vi "Playground.vi"(11 "Inset":refnum<class "Inset.lvclass">) -> (3 "Inset out":refnum<class "Inset.lvclass">)   [LabVIEW 2019, in "Inset.lvclass"]
uses:
  Inset.lvclass
  Parse/Image/SVGImage.lvclass
  C:/Users/Albro/Documents/GitHub/AFM-Lithography/lvsrc/Classes/Parse/SVG Object/SVG Object.lvclass
  Parse/ParseXML/ParseSVG.lvclass
  Parse/ParseVectorFile/ParseVectorFile.lvclass
  Parse/ParseXML/Image.ctl
  Parse/ParseXML/ParseSVG.lvclass/ParseSVG.ctl
  <vilib>/LabVIEW Open Source Project/OpenURI/utilities/isHEXDigit.vi
  BigMAQ/BigMAQ.lvclass
  Parse/EditSVG/EditSVG.lvclass
  <vilib>/LabVIEW Open Source Project/OpenURI/openURI.lvlib
panel:
  out "Pct-Encoded String":string
  out "Edited XML":string
  out "BGD Size":dbl
  out "Y Offset 2":string
  out "ScanSize 2":string
  out "BGD Y Offset":dbl
  out "BGD X Offset":dbl
  out "Inset X Offset":dbl
  out "Inset Y Offset":dbl
  out "Inset Size":dbl
  out "SVGImage.lvclass":refnum<class "SVGImage.lvclass">
  out "ScanSize":string
  out "Y Offset":string
  in  "Inkscape Path":path
  in  "Background Path":path=path "C:/Users/Albro/Documents/GitHub/AFM-Lithography/test files/Inset Test Files/R_tMLG_Au0003.ibw"
  in  "Inset Path":path=path "C:/Users/Albro/Documents/GitHub/AFM-Lithography/test files/Inset Test Files/R_tMLG_Au0004.ibw"
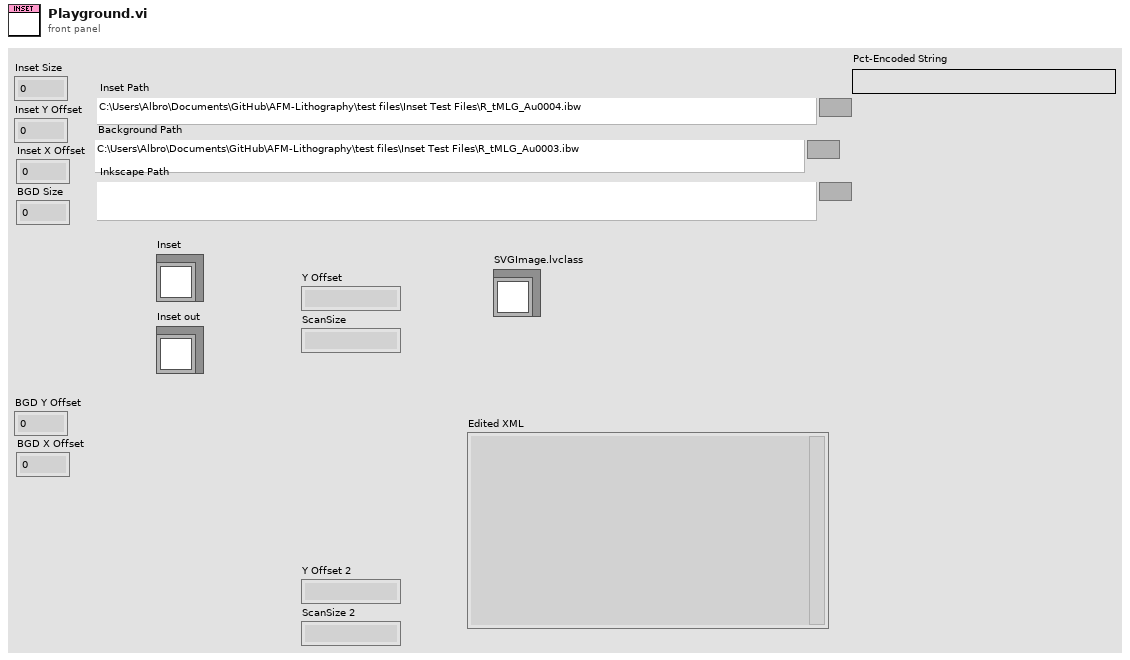
[diagram p1: front panel]
types:
  T1 = cluster{"Inkscape":path, "Background":path, "Inset":path}
  T2 = typedef "ParseSVG.lvclass/Image.ctl" = cluster{"x":string, "y":string, "width":string, "height":string, "xlink:href":string, "id":string, "transform":string}
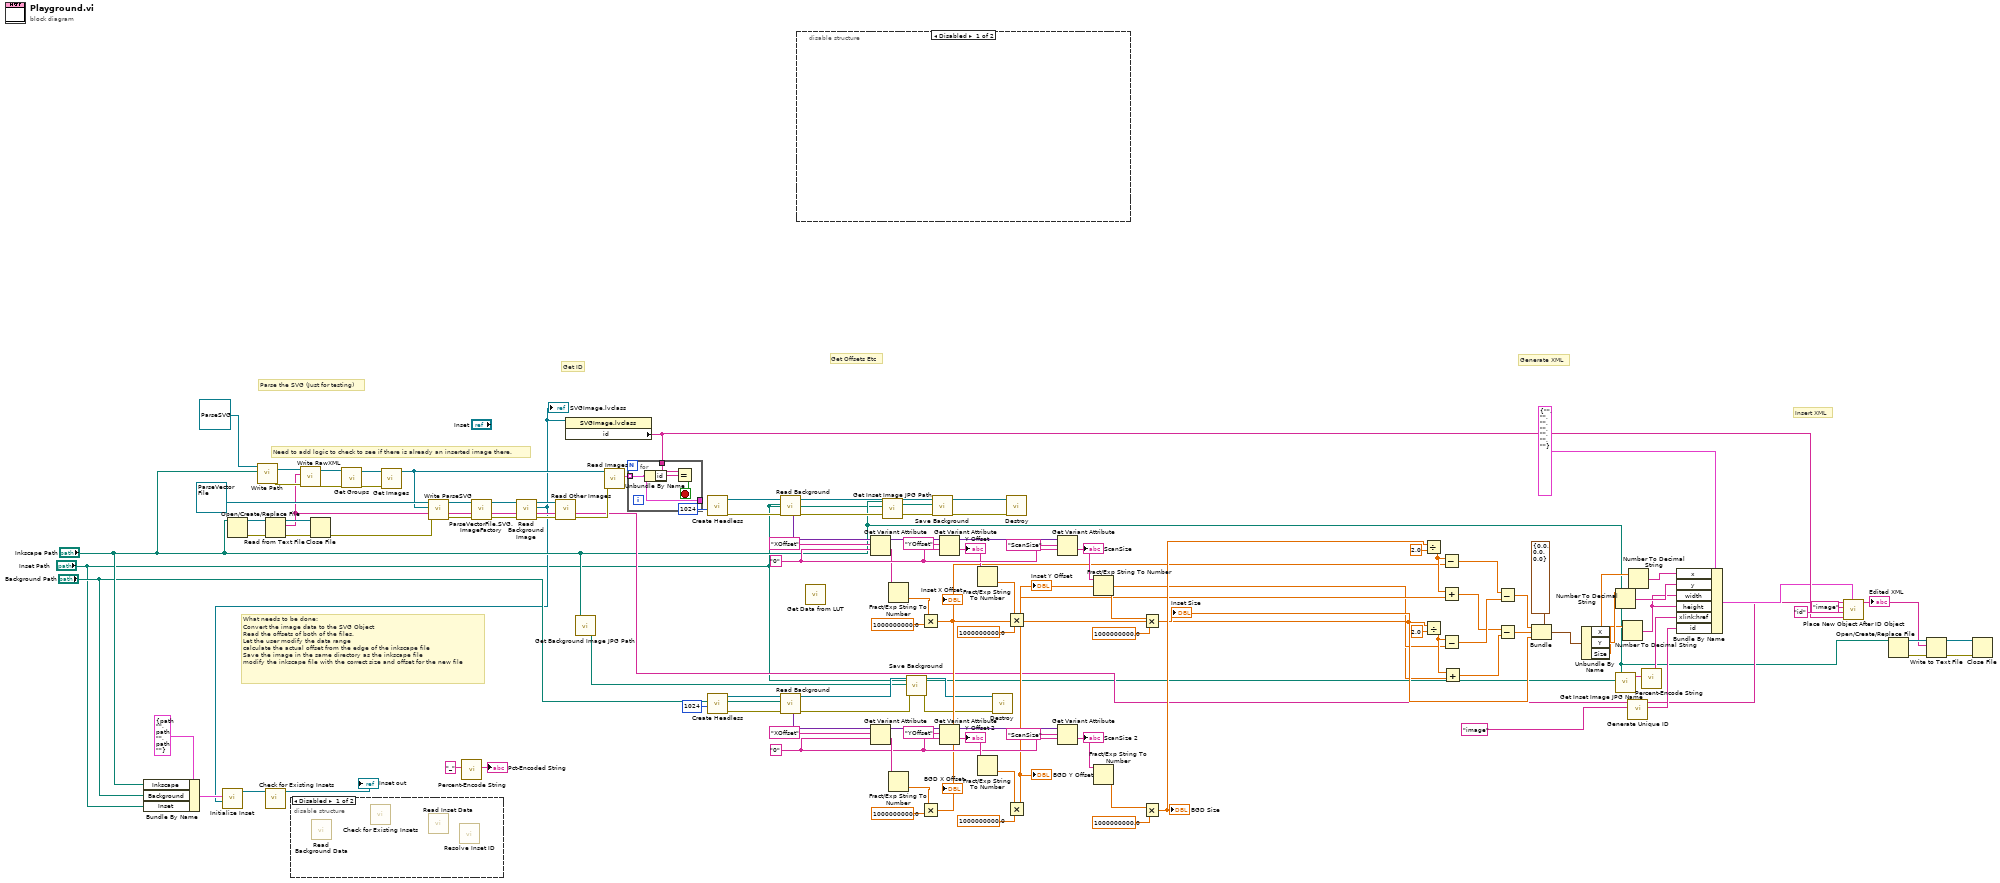
[diagram p0: block diagram]
diagram:
  w66 = "0"
  w114 = "0"
  # "Parse the SVG (Just for testing)"
  # "Insert XML"
  # "Generate XML"
  # "Get Offsets Etc"
  # "Get ID"
  # "Need to add logic to check to see if there is already an inserted image there."
  # "What needs to be done:\nConvert the image data to the SVG Object\nRead the offsets of both of the files.\nLet the user modify the data range\ncalculate the actual offset from the edge of the inkscape file\nSave the image in the same directory as the inkscape file\nmodify the inkscape file with the correct size and offset for the new file"
  n1 = Bundle By Name(cluster=T1 {"Inkscape"=path "", "Background"=path "", "Inset"=path ""} ("Paths"), "Inkscape"="Inkscape Path", "Background"="Background Path", "Inset"="Inset Path") -> (w11:T1)
  n2 = Open/Create/Replace File(file path (use dialog)="Inkscape Path") -> (refnum out=w103:refnum<file>, error out=w101:errorcluster)  [unwired: 5 in, 1 out]
  n3 = call-dynamic "Write Path.vi"("Path"="Inkscape Path", "ParseSVG in"=refnum<class "ParseSVG.lvclass"> refnum) -> ("error out"=w111:errorcluster, "ParseSVG out"=w112:refnum<class "ParseSVG.lvclass">)  [unwired: 8 in]
  n4 = Read from Text File(file (use dialog)=w103, error in=w101) -> (refnum out=w102:refnum<file>, text=w17:string, error out=w100:errorcluster)  [unwired: 2 in, 1 out]
  n5 = disable-structure shown="Disabled" {
    frame Disabled {
      n6 = call "Read Background Data.vi"() -> ()  [unwired: 10 in, 2 out]
      n7 = call "Check for Existing Insets.vi"() -> ()  [unwired: 10 in, 2 out]
      n8 = call "Read Inset Data.vi"() -> ()  [unwired: 10 in, 2 out]
      n9 = call "Resolve Inset ID.vi"() -> ()  [unwired: 10 in, 2 out]
    }
    frame Enabled {
    }
  }
  n10 = call "Write RawXML.vi"("error in (no error)"=w111, "RawXML"=w17, "ParseSVG.lvclass"=w112) -> ("error out"=w109:errorcluster, "ParseSVG.lvclass 2"=w110:refnum<class "ParseSVG.lvclass">)  [unwired: 7 in]
  n11 = Close File(refnum=w102, error in=w100) -> (error out=w99:errorcluster)  [unwired: 1 out]
  n12 = call "Get Groups.vi"("error in (no error)"=w109, "ParseSVG in"=w110) -> ("error out"=w107:errorcluster, "ParseSVG out"=w108:refnum<class "ParseSVG.lvclass">)  [unwired: 8 in]
  n13 = call "Get Images.vi"("error in (no error)"=w107, "ParseSVG in"=w108) -> ("ParseSVG out"=w93:refnum<class "ParseSVG.lvclass">)  [unwired: 8 in, 1 out]
  n14 = call-dynamic "Write ParseSVG.vi"("error in (no error)"=w99, "ParseSVG.lvclass"=w93, "ParseVectorFile in"=refnum<class "ParseVectorFile.lvclass"> refnum ("ParseVectorFile.lvclass")) -> ("error out"=w104:errorcluster, "ParseVectorFile out"=w105:refnum<class "ParseVectorFile.lvclass">)  [unwired: 7 in]
  n15 = call <vilib>:"Percent-Encode String.vi"("String"="_") -> ("Pct-Encoded String"=→"Pct-Encoded String":string)  [unwired: 10 in]
  n16 = call "ParseVectorFile.SVG.ImageFactory.vi"("error in (no error)"=w104, "ParseVectorFile in"=w105) -> ("error out"=w97:errorcluster, "ParseVectorFile out"=w98:refnum<class "ParseVectorFile.lvclass">)  [unwired: 8 in]
  n17 = call-dynamic "Read Background Image.vi"("error in (no error)"=w97, "ParseVectorFile in"=w98) -> ("error out"=w95:errorcluster, "SVGImage.lvclass"=w8:refnum<class "SVGImage.lvclass">, "ParseVectorFile out"=w96:refnum<class "ParseVectorFile.lvclass">)  [unwired: 7 in]
  "SVGImage.lvclass" <- w8
  n18 = call "Initialize Inset.vi"("Background Image"=w8, "Paths"=w11) -> ("Inset out"=w4:refnum<class "Inset.lvclass">)  [unwired: 8 in, 1 out]
  n19 = call "Check for Existing Insets.vi"("Inset in"=w4) -> ("Inset out"=→"Inset out":refnum<class "Inset.lvclass">)  [unwired: 9 in, 1 out]
  n20 = call-dynamic "Read Other Images.vi"("error in (no error)"=w95, "ParseVectorFile in"=w96) -> ("error out"=w94:errorcluster)  [unwired: 7 in, 2 out]
  n21 = property class="SVGImage.lvclass"(reference=w8) -> ("id"=w26:string)  [unwired: 1 in, 2 out]
  n22 = call "Get Background Image JPG Path.vi"("Inkscape Path"="Inkscape Path") -> ("Background JPG Path"=w13:path)  [unwired: 2 in]
  n23 = call "Read Images.vi"("error in (no error)"=w94, "ParseSVG in"=w93) -> ("Images"=w92:T2[])  [unwired: 7 in, 2 out]
  n24 = for {
    tunnel: w92 -> [w120] mode=indexing
    tunnel: w26 -> [w122]
    tunnel: [w120] -> _
    stop <- w121 stop-if-true
    n25 = Unbundle By Name(w120) -> ("id"=w123:string)
    n26 = Equal?(x=w122, y=w123) -> (x = y?=w121:bool)
  }
  n27 = call "Create Headless.vi"("Resolution"=1024) -> ("error out"=w89:errorcluster, "BigMAQ out"=w90:refnum<class "BigMAQ.lvclass">)  [unwired: 9 in]
  n28 = call "Create Headless.vi"("Resolution"=1024) -> ("error out"=w77:errorcluster, "BigMAQ out"=w78:refnum<class "BigMAQ.lvclass">)  [unwired: 9 in]
  n29 = call "Read Background.vi"("error in (no error)"=w89, "Path"="Inset Path", "BigMAQ in"=w90) -> ("error out"=w56:errorcluster, "BigMAQ out"=w59:refnum<class "BigMAQ.lvclass">, "Metadata"=w88:variant)  [unwired: 6 in]
  n30 = call "Read Background.vi"("error in (no error)"=w77, "Path"="Background Path", "BigMAQ in"=w78) -> ("error out"=w14:errorcluster, "BigMAQ out"=w16:refnum<class "BigMAQ.lvclass">, "Metadata"=w60:variant)  [unwired: 6 in]
  n31 = disable-structure shown="Disabled" {
    frame Disabled {
    }
    frame Enabled {
    }
  }
  n32 = call "Get Data from LUT.vi"() -> ()  [unwired: 9 in, 3 out]
  n33 = Get Variant Attribute(Variant=w88, name="XOffset", default value (empty Variant)=w114) -> (duplicate Variant=w118:variant, value=w85:string)  [unwired: 1 in, 2 out]
  n34 = Get Variant Attribute(Variant=w60, name="XOffset", default value (empty Variant)=w66) -> (duplicate Variant=w62:variant, value=w69:string)  [unwired: 1 in, 2 out]
  n35 = call "Get Inset Image JPG Path.vi"("Inset Data Path"="Inset Path", "Inkscape Path"="Inkscape Path") -> ("Inset JPG Path"=w57:path)  [unwired: 3 in]
  n36 = Fract/Exp String To Number(string=w85) -> (number=w84:dbl)  [unwired: 3 in, 1 out]
  n37 = Fract/Exp String To Number(string=w69) -> (number=w70:dbl)  [unwired: 3 in, 1 out]
  n38 = call "Save Background.vi"("error in"=w14, "File Path"=w13, "BigMAQ in"=w16) -> ("error out"=w6:errorcluster, "BigMAQ out"=w15:refnum<class "BigMAQ.lvclass">)  [unwired: 7 in]
  n39 = Multiply(x=w84, y=1000000000.0) -> (x*y=w41:dbl)
  "Inset X Offset" <- w41
  n40 = Multiply(x=w70, y=1000000000.0) -> (x*y=w44:dbl)
  "BGD X Offset" <- w44
  n41 = call "Save Background.vi"("error in"=w56, "File Path"=w57, "BigMAQ in"=w59) -> ("error out"=w7:errorcluster, "BigMAQ out"=w58:refnum<class "BigMAQ.lvclass">)  [unwired: 7 in]
  n42 = Get Variant Attribute(Variant=w118, name="YOffset", default value (empty Variant)=w114) -> (duplicate Variant=w116:variant, value=w86:string)  [unwired: 1 in, 2 out]
  "Y Offset" <- w86
  n43 = Get Variant Attribute(Variant=w62, name="YOffset", default value (empty Variant)=w66) -> (duplicate Variant=w64:variant, value=w68:string)  [unwired: 1 in, 2 out]
  "Y Offset 2" <- w68
  n44 = Fract/Exp String To Number(string=w86) -> (number=w81:dbl)  [unwired: 3 in, 1 out]
  n45 = Fract/Exp String To Number(string=w68) -> (number=w73:dbl)  [unwired: 3 in, 1 out]
  n46 = call "Destroy.vi"("error in"=w6, "BigMAQ in"=w15) -> ()  [unwired: 8 in, 2 out]
  n47 = call "Destroy.vi"("error in"=w7, "BigMAQ in"=w58) -> ()  [unwired: 8 in, 2 out]
  n48 = Multiply(x=w81, y=1000000000.0) -> (x*y=w40:dbl)
  "Inset Y Offset" <- w40
  n49 = Multiply(x=w73, y=1000000000.0) -> (x*y=w43:dbl)
  "BGD Y Offset" <- w43
  n50 = Get Variant Attribute(Variant=w116, name="ScanSize", default value (empty Variant)=w114) -> (value=w87:string)  [unwired: 1 in, 3 out]
  "ScanSize" <- w87
  n51 = Get Variant Attribute(Variant=w64, name="ScanSize", default value (empty Variant)=w66) -> (value=w67:string)  [unwired: 1 in, 3 out]
  "ScanSize 2" <- w67
  n52 = Fract/Exp String To Number(string=w87) -> (number=w79:dbl)  [unwired: 3 in, 1 out]
  n53 = Fract/Exp String To Number(string=w67) -> (number=w75:dbl)  [unwired: 3 in, 1 out]
  n54 = Multiply(x=w79, y=1000000000.0) -> (x*y=w42:dbl)
  "Inset Size" <- w42
  n55 = Multiply(x=w75, y=1000000000.0) -> (x*y=w45:dbl)
  "BGD Size" <- w45
  n56 = Divide(x=w45, y=2.0) -> (x/y=w54:dbl)
  n57 = Divide(x=w42, y=2.0) -> (x/y=w53:dbl)
  n58 = Subtract(x=w54, y=w44) -> (x-y=w51:dbl)
  n59 = Add(x=w54, y=w43) -> (x+y=w49:dbl)
  n60 = Subtract(x=w53, y=w41) -> (x-y=w50:dbl)
  n61 = Add(x=w53, y=w40) -> (x+y=w48:dbl)
  n62 = Subtract(x=w51, y=w50) -> (x-y=w46:dbl)
  n63 = Subtract(x=w49, y=w48) -> (x-y=w47:dbl)
  n64 = Bundle(cluster=cluster{"X":dbl, "Y":dbl, "Size":dbl} {"X"=0.0, "Y"=0.0, "Size"=0.0}, "X"=w46, "Y"=w47, "Size"=w42) -> (w37:cluster{"X":dbl, "Y":dbl, "Size":dbl})
  n65 = Unbundle By Name(w37) -> ("X"=w36:dbl, "Y"=w34:dbl, "Size"=w32:dbl)
  n66 = Number To Decimal String(number=w34) -> (decimal integer string=w33:string)  [unwired: 1 in]
  n67 = call "Get Inset Image JPG Name.vi"("Inset Data Path"="Inset Path", "Inkscape Path"="Inkscape Path") -> ("Inset JPG Name"=w24:string)  [unwired: 3 in]
  n68 = Number To Decimal String(number=w32) -> (decimal integer string=w31:string)  [unwired: 1 in]
  n69 = call "Generate Unique ID.vi"("Basename"="image", "XML String"=w17) -> ("Unique ID"=w30:string)  [unwired: 9 in]
  n70 = Number To Decimal String(number=w36) -> (decimal integer string=w35:string)  [unwired: 1 in]
  n71 = call <vilib>:"Percent-Encode String.vi"("String"=w24) -> ("Pct-Encoded String"=w23:string)  [unwired: 10 in]
  n72 = Bundle By Name(cluster=T2 {"x"="", "y"="", "width"="", "height"="", "xlink:href"="", "id"="", "transform"=""} ("image"), "x"=w35, "y"=w33, "width"=w31, "height"=w31, "xlink:href"=w23, "id"=w30) -> (w25:T2)
  n73 = call "Place New Object After ID Object.vi"("Named Cluster"=w25, "Identifying Attribute Value"=w26, "Identifying Attribute Type"="id", "Element Type"="image", "XML String"=w17) -> ("Edited XML"=w18:string)  [unwired: 6 in]
  "Edited XML" <- w18
  n74 = Open/Create/Replace File(file path (use dialog)="Inkscape Path") -> (refnum out=w20:refnum<file>, error out=w22:errorcluster)  [unwired: 5 in, 1 out]
  n75 = Write to Text File(file (use dialog)=w20, text=w18, error in=w22) -> (refnum out=w19:refnum<file>, error out=w21:errorcluster)  [unwired: 1 in, 1 out]
  n76 = Close File(refnum=w19, error in=w21) -> ()  [unwired: 2 out]
